vi "SaveGageData.vi"(4 "Keep array":T1(array[cluster]), 5 "TGC data":i16[][][](array[numeric]), 6 "folder path":path=path "D:/Temp", 7 "Data":i16[][][][](array[numeric]), 8 "operator":string, 9 "ID":i32, 10 "Array":T3[](array[typedef]) {"Compression Parameters"."% taper" min=50 max=1000 format="%.2f"; "Compression Parameters"."F2 (MHz)" format="%.3f"; "Compression Parameters"."F1 (MHz)" format="%.3f"; "Scan Settings"."prf (kHz)" format="%.2f"; "Therapy Parameters"."Therapy amplitude (mV)" min=50 max=1000 format="%.2f"; "Therapy Parameters"."Time on (s)" format="%.3f"; "Therapy Parameters"."Theraputic Freq (MHz)" format="%.3f"; "Patient Info"."Race" items=["Am Ind or Alaska", "Asian", "Hawaiian, Pac Isl", "Black or Afr Amer", "White", "more than one race", "unknown"]; "Patient Info"."Ethnicty 2" items=["Hispanic", "Non-Hispanic", "unknown"]; "Patient Info"."LOS" items=["1", "2", "3", "4", "5"]; "Patient Info"."PSA" format="%.1f"; "Scan Info"."delay" format="%.2f"; "Scan Info"."pivot distance" format="%.2f"; "Scan Info"."sector scan angle" format="%.2f"; "Tranducer Info"."bandwidth" format="%.2f"; "Tranducer Info"."center freq" format="%.2f"; "Tranducer Info"."start freq" format="%.2f"}, 11 "Machine Params":T2 {"Scan Info"."sector scan angle" format="%.2f"; "Scan Info"."pivot distance" format="%.2f"; "Scan Info"."delay" format="%.2f"}) -> ()   [LabVIEW 2022 SP3]
uses:
  ViewData/-ReadEye/Header.ctl
  MachineParams.ctl
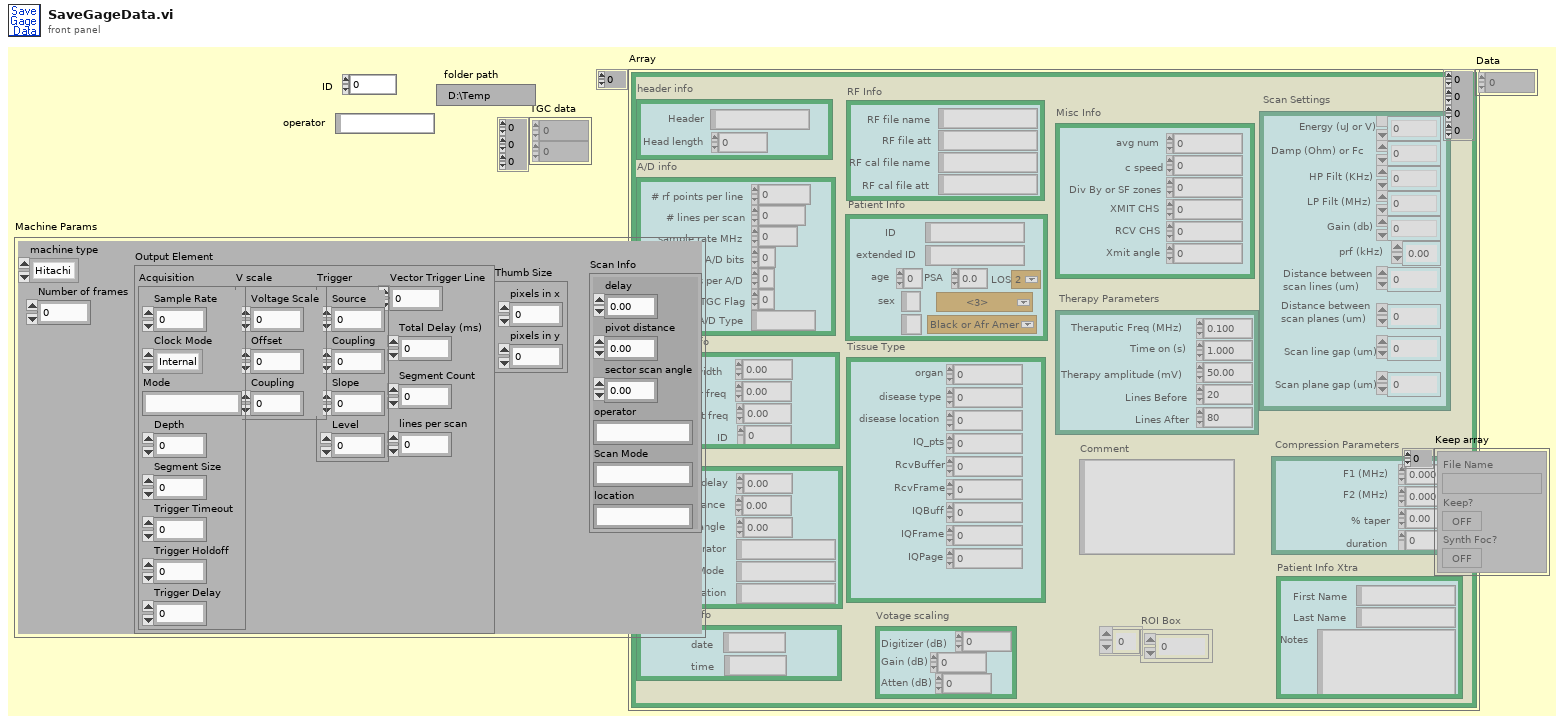
[diagram p1: front panel]
types:
  T1 = cluster{"File Name":string, "Keep?":bool, "Synth Foc?":bool}[]
  T2 = typedef "MachineParams.ctl" = cluster{"machine type":enum16{"Hitachi", "B&K 3535", "B&K Hawk"}, "Number of frames":dbl, "Output Element":cluster{"Acquisition":cluster{"Sample Rate":dbl, "Clock Mode":enum16{"Internal", "External", "Reference"}, "Mode":string, "Depth":dbl, "Segment Size":dbl, "Trigger Timeout":dbl, "Trigger Holdoff":dbl, "Trigger Delay":dbl}, "V scale":cluster{"Voltage Scale":i16, "Offset":dbl, "Coupling":u16}, "Trigger":cluster{"Source":u16, "Coupling":u16, "Slope":u16, "Level":dbl}, "Vector Trigger Line":i16, "Total Delay (ms)":dbl, "Segment Count":u32, "lines per scan":i32}, "Thumb Size":cluster{"pixels in x":i16, "pixels in y":i16}, "Scan Info":cluster{"delay":sgl, "pivot distance":sgl, "sector scan angle":sgl, "operator":string, "Scan Mode":string, "location":string}}
  T3 = typedef "Header.ctl" = cluster{"header info":cluster{"Header":string, "Head length":i16}, "A/D info":cluster{"# rf points per line":u16, "# lines per scan":u16, "sample rate MHz":u16, "# A/D bits":i16, "# bytes per A/D":u16, "TGC Flag":u16, "A/D Type":string}, "Tranducer Info":cluster{"bandwidth":sgl, "center freq":sgl, "start freq":sgl, "ID":i32}, "Scan Info":cluster{"delay":sgl, "pivot distance":sgl, "sector scan angle":sgl, "operator":string, "Scan Mode":string, "location":string}, "Time/Date Info":cluster{"date":string, "time":string}, "RF Info":cluster{"RF file name":string, "RF file att":string, "RF cal file name":string, "RF cal file att":string}, "Patient Info":cluster{"ID":string, "extended ID":string, "age":u16, "sex":string, "previously\nscanned":string, "PSA":sgl, "LOS":u8, "Ethnicty 2":u8, "Race":u8}, "Tissue Type":cluster{"organ":i16, "disease type":i16, "disease location":i16, "IQ_pts":u16, "RcvBuffer":u8, "RcvFrame":u16, "IQBuff":u8, "IQFrame":u16, "IQPage":u8}, "Votage scaling":cluster{"Digitizer (dB)":sgl, "Gain (dB)":sgl, "Atten (dB)":sgl}, "Comment":string, "Misc Info":cluster{"avg num":u16, "c speed":i16, "Div By or SF zones":i16, "XMIT CHS":u8, "RCV CHS":u8, "Xmit angle":sgl}, "Therapy Parameters":cluster{"Theraputic Freq (MHz)":sgl, "Time on (s)":sgl, "Therapy amplitude (mV)":sgl, "Lines Before":u16, "Lines After":u16}, "Scan Settings":cluster{"Energy (uJ or V)":u8, "Damp (Ohm) or Fc":u8, "HP Filt (KHz)":u8, "LP Filt (MHz)":u8, "Gain (db)":u8, "prf (kHz)":sgl, "Distance between\nscan lines (um)":u16, "Distance between\nscan planes (um)":u16, "Scan line gap (um)":sgl, "Scan plane gap (um)":sgl}, "Compression Parameters":cluster{"F1 (MHz)":sgl, "F2 (MHz)":sgl, "% taper":sgl, "duration":sgl}, "Patient Info Xtra":cluster{"First Name":string, "Last Name":string, "Notes":string}, "ROI Box":u16[]}
  T4 = enum16{"big-endian, network order", "native, host order", "little-endian"}
  T5 = enum16{"open", "replace", "create", "open or create", "replace or create", "replace or create with confirmation"}
  T6 = cluster{"bandwidth":sgl, "center freq":sgl, "start freq":sgl, "ID":i32}
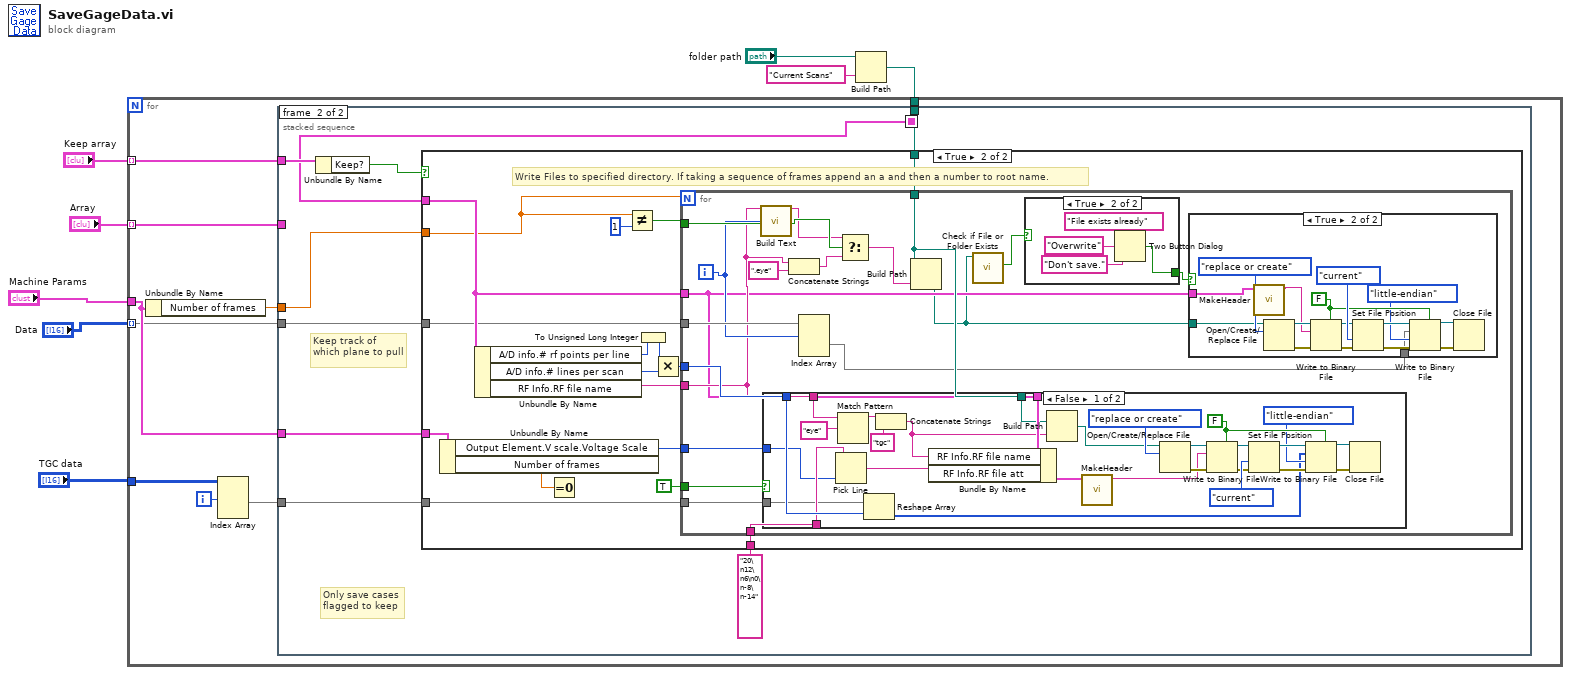
[diagram p0: block diagram]
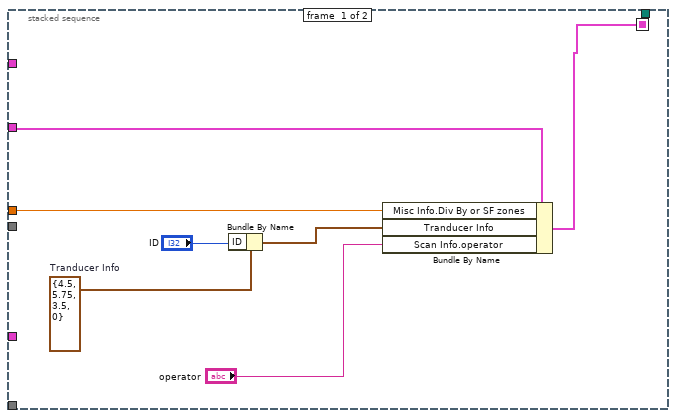
[diagram p2: hidden frame]
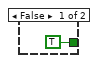
[diagram p4: hidden frame]
diagram:
  n1 = Build Path(base path="folder path", name or relative path="Current Scans") -> (appended path=w6:path)
  n2 = for {
    tunnel: "Array" -> [w13] mode=indexing
    tunnel: "TGC data" -> [w17]
    tunnel: w6 -> [w16]
    tunnel: "Keep array" -> [w12] mode=indexing
    tunnel: "Machine Params" -> [w10]
    tunnel: "Data" -> [w9] mode=indexing
    i -> [w14]
    n3 = Unbundle By Name(w10) -> ("Number of frames"=w11:dbl)
    n4 = Index Array(array=w17, index (dim 0)=w14) -> (element=w15:i16[][])  [unwired: 2 in]
    n5 = stacked-sequence {
      seq-local: [w24 _] -> [_ w28]
      tunnel: w13 -> [w20 _]
      tunnel: w15 -> [_ w32]
      tunnel: w16 -> [_ w31]
      tunnel: w12 -> [_ w29]
      tunnel: w11 -> [w19 w27]
      tunnel: w10 -> [_ w26]
      tunnel: w9 -> [_ w25]
      frame #0 {
        w23 = T6 {"bandwidth"=4.5, "center freq"=5.75, "start freq"=3.5, "ID"=0}  # Tranducer Info
        n6 = Bundle By Name(cluster=w23, "ID"="ID") -> (w21:T6)
        n7 = Bundle By Name(cluster=w20, "Misc Info.Div By or SF zones"=w19, "Tranducer Info"=w21, "Scan Info.operator"="operator") -> (w24:T3)
      }
      frame #1 {
        # "Keep track of which plane to pull"
        # "Only save cases\nflagged to keep"
        n8 = Unbundle By Name(w29) -> ("Keep?"=w33:bool)
        n9 = case shown="True" w33 {
          tunnel: w28 -> [_ w38]
          tunnel: w32 -> [_ w44]
          tunnel: w31 -> [_ w41]
          tunnel: "20\n12\n6\n0\n-8\n-14" -> [_ w40]
          tunnel: w27 -> [_ w37]
          tunnel: w26 -> [_ w36]
          tunnel: w25 -> [_ w34]
          frame False {
          }
          frame True {
            # "Write Files to specified directory. If taking a sequence of frames append an a and then a number to root name."
            n10 = Unbundle By Name(w36) -> ("Output Element.V scale.Voltage Scale"=w39:i16, "Number of frames"=w45:dbl)
            n11 = Unbundle By Name(w38) -> ("A/D info.# rf points per line"=w50:u16, "A/D info.# lines per scan"=w49:u16, "RF Info.RF file name"=w47:string)
            n12 = Equal To 0?(x=w45) -> ()  [unwired: 1 out]
            n13 = Not Equal?(x=w37, y=1) -> (x != y?=w42:bool)
            n14 = To Unsigned Long Integer(number=w50) -> (unsigned 32bit integer=w46:u32)
            n15 = Multiply(x=w46, y=w49) -> (x*y=w48:u32)
            n16 = for {
              N: w37 -> [_]
              tunnel: w34 -> [w61]
              tunnel: w48 -> [w67]
              tunnel: w41 -> [w64]
              tunnel: w47 -> [w57]
              tunnel: w38 -> [w54]
              tunnel: TRUE -> [w69]
              tunnel: w44 -> [w68]
              tunnel: w42 -> [w65]
              tunnel: w40 -> [w63]
              tunnel: w39 -> [w62]
              i -> [w59]
              n17 = call "Build Text"("Beginning Text"=w57, "num"=w59) -> ("Result"=w58:string)  [unwired: 12 in, 1 out]
              n18 = case shown="False" w69 {
                tunnel: w57 -> [w118 _]
                tunnel: w54 -> [w114 _]
                tunnel: w68 -> [w106 _]
                tunnel: w64 -> [w112 _]
                tunnel: w67 -> [w110 _]
                tunnel: w63 -> [w108 _]
                tunnel: w62 -> [w107 _]
                frame False {
                  w96 = FALSE ("prepend array or string size? (T)")
                  n19 = Pick Line(multi-line string=w108, line index=w107) -> (output string=w109:string)  [unwired: 1 out]
                  n20 = Match Pattern(string=w118, regular expression="eye") -> (before substring=w116:string)  [unwired: 4 out]
                  n21 = Reshape Array(w106, w110) -> (w91:i16[])
                  n22 = Concatenate Strings(w116, "tgc") -> (w111:string)
                  n23 = Bundle By Name(cluster=w114, "RF Info.RF file name"=w111, "RF Info.RF file att"=w109) -> (w113:T3)
                  n24 = Build Path(base path=w112, name or relative path=w111) -> (appended path=w93:path)
                  n25 = call "MakeHeader.vi"("Header In"=w113) -> ("Header String"=w92:string)  [unwired: 6 out]
                  n26 = Open/Create/Replace File(file path (use dialog)=w93, operation (0:open)=T5."replace or create") -> (refnum out=w100:refnum<file>, error out=w99:errorcluster)  [unwired: 1 in, 4 out]
                  n27 = Write to Binary File(file (use dialog)=w100, data=w92, error in=w99, 5:w96) -> (refnum out=w102:refnum<file>, error out=w101:errorcluster)  [unwired: 3 out]
                  n28 = Set File Position(refnum=w102, from (0:start)=enum16{"start", "end", "current"}."current" ("pos mode (0:2)"), error in=w101) -> (refnum out=w98:refnum<file>, error out=w97:errorcluster)  [unwired: 1 out]
                  n29 = Write to Binary File(file (use dialog)=w98, data=w91, error in=w97, 5:w96, 9:T4."little-endian" ("byte order (0:big-endian, network order)")) -> (refnum out=w104:refnum<file>, error out=w105:errorcluster)  [unwired: 2 out]
                  n30 = Close File(refnum=w104, error in=w105) -> ()  [unwired: 2 out]
                }
                frame True {
                }
              }
              n31 = Concatenate Strings(w57, ".eye" ("string")) -> (w55:string)
              n32 = Index Array(array=w61, index (dim 0)=w59) -> (element=w60:i16[][])  [unwired: 2 in]
              n33 = Select(t=w58, s=w65, f=w55) -> (s? t:f=w66:string)
              n34 = Build Path(base path=w64, name or relative path=w66) -> (appended path=w53:path)
              n35 = call <vilib>:"Check if File or Folder Exists.vi"("path"=w53) -> ("file or folder exists?"=w52:bool)  [unwired: 8 in, 2 out]
              n36 = case shown="True" w52 {
                tunnel: [TRUE ("T button?") w71] -> w51
                frame False {
                }
                frame True {
                  n37 = Two Button Dialog(message="File exists already", 1:"Don't save." ("F button name (\"Cancel\")"), 2:"Overwrite" ("T button name (\"OK\")")) -> (T button?=w71:bool)
                }
              }
              n38 = case shown="True" w51 {
                tunnel: w60 -> [_ w78]
                tunnel: w54 -> [_ w76]
                tunnel: w53 -> [_ w75]
                frame False {
                }
                frame True {
                  w80 = FALSE ("prepend array or string size? (T)")
                  n39 = call "MakeHeader.vi"("Header In"=w76) -> ("Header String"=w77:string)  [unwired: 6 out]
                  n40 = Open/Create/Replace File(file path (use dialog)=w75, operation (0:open)=T5."replace or create") -> (refnum out=w84:refnum<file>, error out=w83:errorcluster)  [unwired: 1 in, 4 out]
                  n41 = Write to Binary File(file (use dialog)=w84, data=w77, error in=w83, 5:w80) -> (refnum out=w86:refnum<file>, error out=w85:errorcluster)  [unwired: 3 out]
                  n42 = Set File Position(refnum=w86, from (0:start)=enum16{"start", "end", "current"}."current" ("pos mode (0:2)"), error in=w85) -> (refnum out=w82:refnum<file>, error out=w81:errorcluster)  [unwired: 1 out]
                  n43 = Write to Binary File(file (use dialog)=w82, data=w78, error in=w81, 5:w80, 9:T4."little-endian" ("byte order (0:big-endian, network order)")) -> (refnum out=w88:refnum<file>, error out=w89:errorcluster)  [unwired: 2 out]
                  n44 = Close File(refnum=w88, error in=w89) -> ()  [unwired: 2 out]
                }
              }
            }
          }
        }
      }
    }
  }
